vi "Agilent DSO1000 Series Acquire Waveform Continuously.vi"() -> ()   [LabVIEW 2010]
doc: "This example shows how to use autosetup and acquire a waveform continuously on a single channel.\n In this example, each record is acquired independently and not as a continuous stream of data."
uses:
  <instrlib>/Agilent DSO1000 Series/Public/Data/Read Waveform (Single).vi
  <instrlib>/Agilent DSO1000 Series/Agilent DSO1000 Series.lvlib
panel:
  in  "Channel (1: Channel 1)":u16(ring)=1 items=["Channel 1"=1, "Channel 2"=2, "Channel 3"=3, "Channel 4"=4]
  in  "Maximum Time (10000 ms)":u32=10000
  in  "stop":bool
  in  "Probe Attenuation (10.0)":dbl=10.0
  out "Waveform Data":waveform(dbl)(graph)
  in  "VISA resource name":refnum<visa-resource-name>
  # "(c) 2009 National Instruments.  ALL RIGHTS RESERVED."
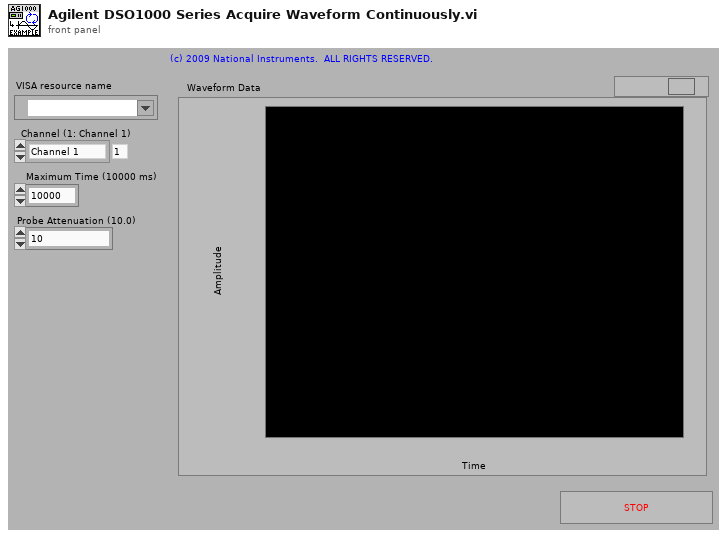
[diagram p1: front panel]
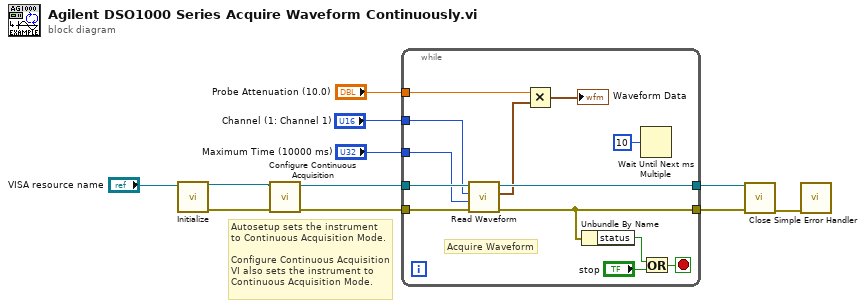
[diagram p0: block diagram]
diagram:
  # "Autosetup sets the instrument\nto Continuous Acquisition Mode.\n\nConfigure Continuous Acquisition VI also sets the instrument to Continuous Acquisition Mode."
  n1 = call <instrlib>:"Initialize.vi"("VISA resource name"="VISA resource name") -> ("error out"=w4:errorcluster, "VISA resource name out"=w6:refnum<visa-resource-name>)  [unwired: 9 in]
  n2 = call <instrlib>:"Configure Continuous Acquisition.vi"("error in (no error)"=w4, "VISA resource name"=w6) -> ("error out"=w3:errorcluster, "VISA resource name out"=w5:refnum<visa-resource-name>)  [unwired: 8 in]
  n3 = while {
    tunnel: w5 -> [w18]
    tunnel: w3 -> [w14]
    tunnel: [w17] -> w2
    tunnel: [w13] -> w1
    tunnel: "Channel (1: Channel 1)" -> [w12]
    tunnel: "Probe Attenuation (10.0)" -> [w24]
    tunnel: "Maximum Time (10000 ms)" -> [w15]
    stop <- w21 stop-if-true
    # "Acquire Waveform"
    n4 = call-poly <instrlib>:"Read Waveform.vi"("error in (no error)"=w14, "Maximum Time (10000 ms)"=w15, "Channel (1: Channel 1)"=w12, "VISA resource name"=w18) -> ("error out"=w13:errorcluster, "Waveform Data"=w16:waveform(dbl), "VISA resource name out"=w17:refnum<visa-resource-name>)  [unwired: 5 in]
    n5 = Multiply(x=w24, y=w16) -> (x*y=→"Waveform Data":waveform(dbl))
    n6 = Unbundle By Name(w13) -> ("status"=w20:bool)
    n7 = Wait Until Next ms Multiple(millisecond multiple=u32 10) -> ()  [unwired: 1 out]
    n8 = Or(x=w20, y="stop") -> (x .or. y?=w21:bool)
  }
  n9 = call <instrlib>:"Close.vi"("error in (no error)"=w1, "VISA resource name"=w2) -> ("error out"=w11:errorcluster)  [unwired: 9 in]
  n10 = call <vilib>:"Simple Error Handler.vi"("error in (no error)"=w11) -> ()  [unwired: 4 in, 5 out]
